vi "Depth Parser.vi"(8 "error in (no error)":errorcluster, 10 "RDS Serial Frame":refnum<class "RDS Serial Frame.lvclass">, 11 "Depth Instrument in":refnum<class "Depth Instrument.lvclass">) -> (0 "error out":errorcluster, 3 "Depth Instrument out":refnum<class "Depth Instrument.lvclass">)   [LabVIEW 2015, in "Depth Instrument.lvlib" / "Depth Instrument.lvclass"]
uses:
  Depth Instrument.lvclass
  Libraries/RDS Serial Handler/RDS Serial Frame.lvclass
  Libraries/RDS Child Messages/AIP Status Message/AIP Status Response.lvclass
  Libraries/RDS Instruments/AIP/AIP Status.ctl
  Libraries/RDS Instruments/AIP/AIP States.ctl
  Libraries/RDS Serial Handler/RDS Serial Frame.lvclass/RDS Serial Frame.ctl
  Libraries/RDS Framework/RDS Message ID.ctl
  Libraries/RDS Child Messages/Depth Data Message/Depth Data Message.lvclass
  Libraries/RDS Child Messages/Depth Data Message/Depth Data.ctl
  Depth Instrument.lvclass/Depth Instrument.ctl
  Libraries/RDS Framework/RDS Message Class/RDS Message.lvclass/RDS Message.ctl
  Libraries/RDS Child Messages/Depth Data Message/Depth Data Message.lvclass/Depth Data Message.ctl
  Libraries/RDS Serial Handler/RDS Serial Handler.lvlib
  Libraries/RDS Instruments/RDS Instrument Library.lvlib
  Libraries/RDS Child Messages/RDS Child Messages.lvlib
  AIP Instrument/AIP Instrument/AIP Instrument.lvclass
  Libraries/RDS Framework/RDS Message Class/RDS Message.lvclass
  Actors/RDS Parent Actor/RDS Parent Actor/RDS Parent Actor.lvclass
panel:
  out "AIP State":T1
  out "AIP Status Response":refnum<class "AIP Status Response.lvclass">
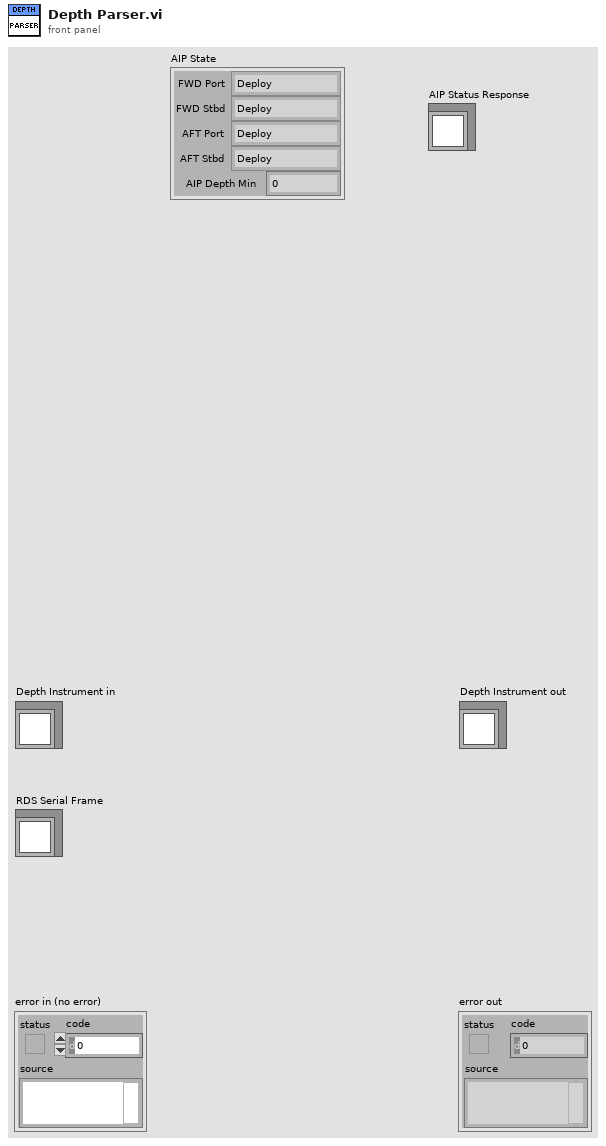
[diagram p1: front panel]
types:
  T1 = typedef "RDS Instrument Library.lvlib/AIP Status.ctl" = cluster{"FWD Port":T2, "FWD Stbd":T2, "AFT Port":T2, "AFT Stbd":T2, "AIP Depth Min":u8}
  T2 = typedef "RDS Instrument Library.lvlib/AIP States.ctl" = enum16{"Deploy", "Deploying", "Deployed", "Stow", "Stowing", "Stowed", "Fault", "brakeOnStow", "breakOnDeploy", "Stopped", "Stopping"}
  T3 = typedef "RDS Child Messages.lvlib/Depth Data.ctl" = cluster{"Depth":sgl, "Water Temp":i8}
  T4 = typedef "RDS Child Messages.lvlib/RDS Message ID.ctl" = enum16{"RDS Hello World", "String Message", "AIP_Status", "AIP_Command", "GPS_Data", "MCB_Command", "MCB_Status", "Compass_Data", "Depth_Data", "Battery_Data", "Contoller_State", "Set_Mag_Dev", "BTB_Shutdown", "State_Sample_Request", "State_Sample", "PID_Gains_Set", "Helm_Limiter_Set", "Helm_Heading_Command", "Helm_Steering_Command", "Helm_Status", "Controller_Message", "AIP_Set_Min_Depth", "Mission_Controller_State", "Mission_Upload", "Mission_Set_Op_and_Run", "Mission_Settings_Set"}
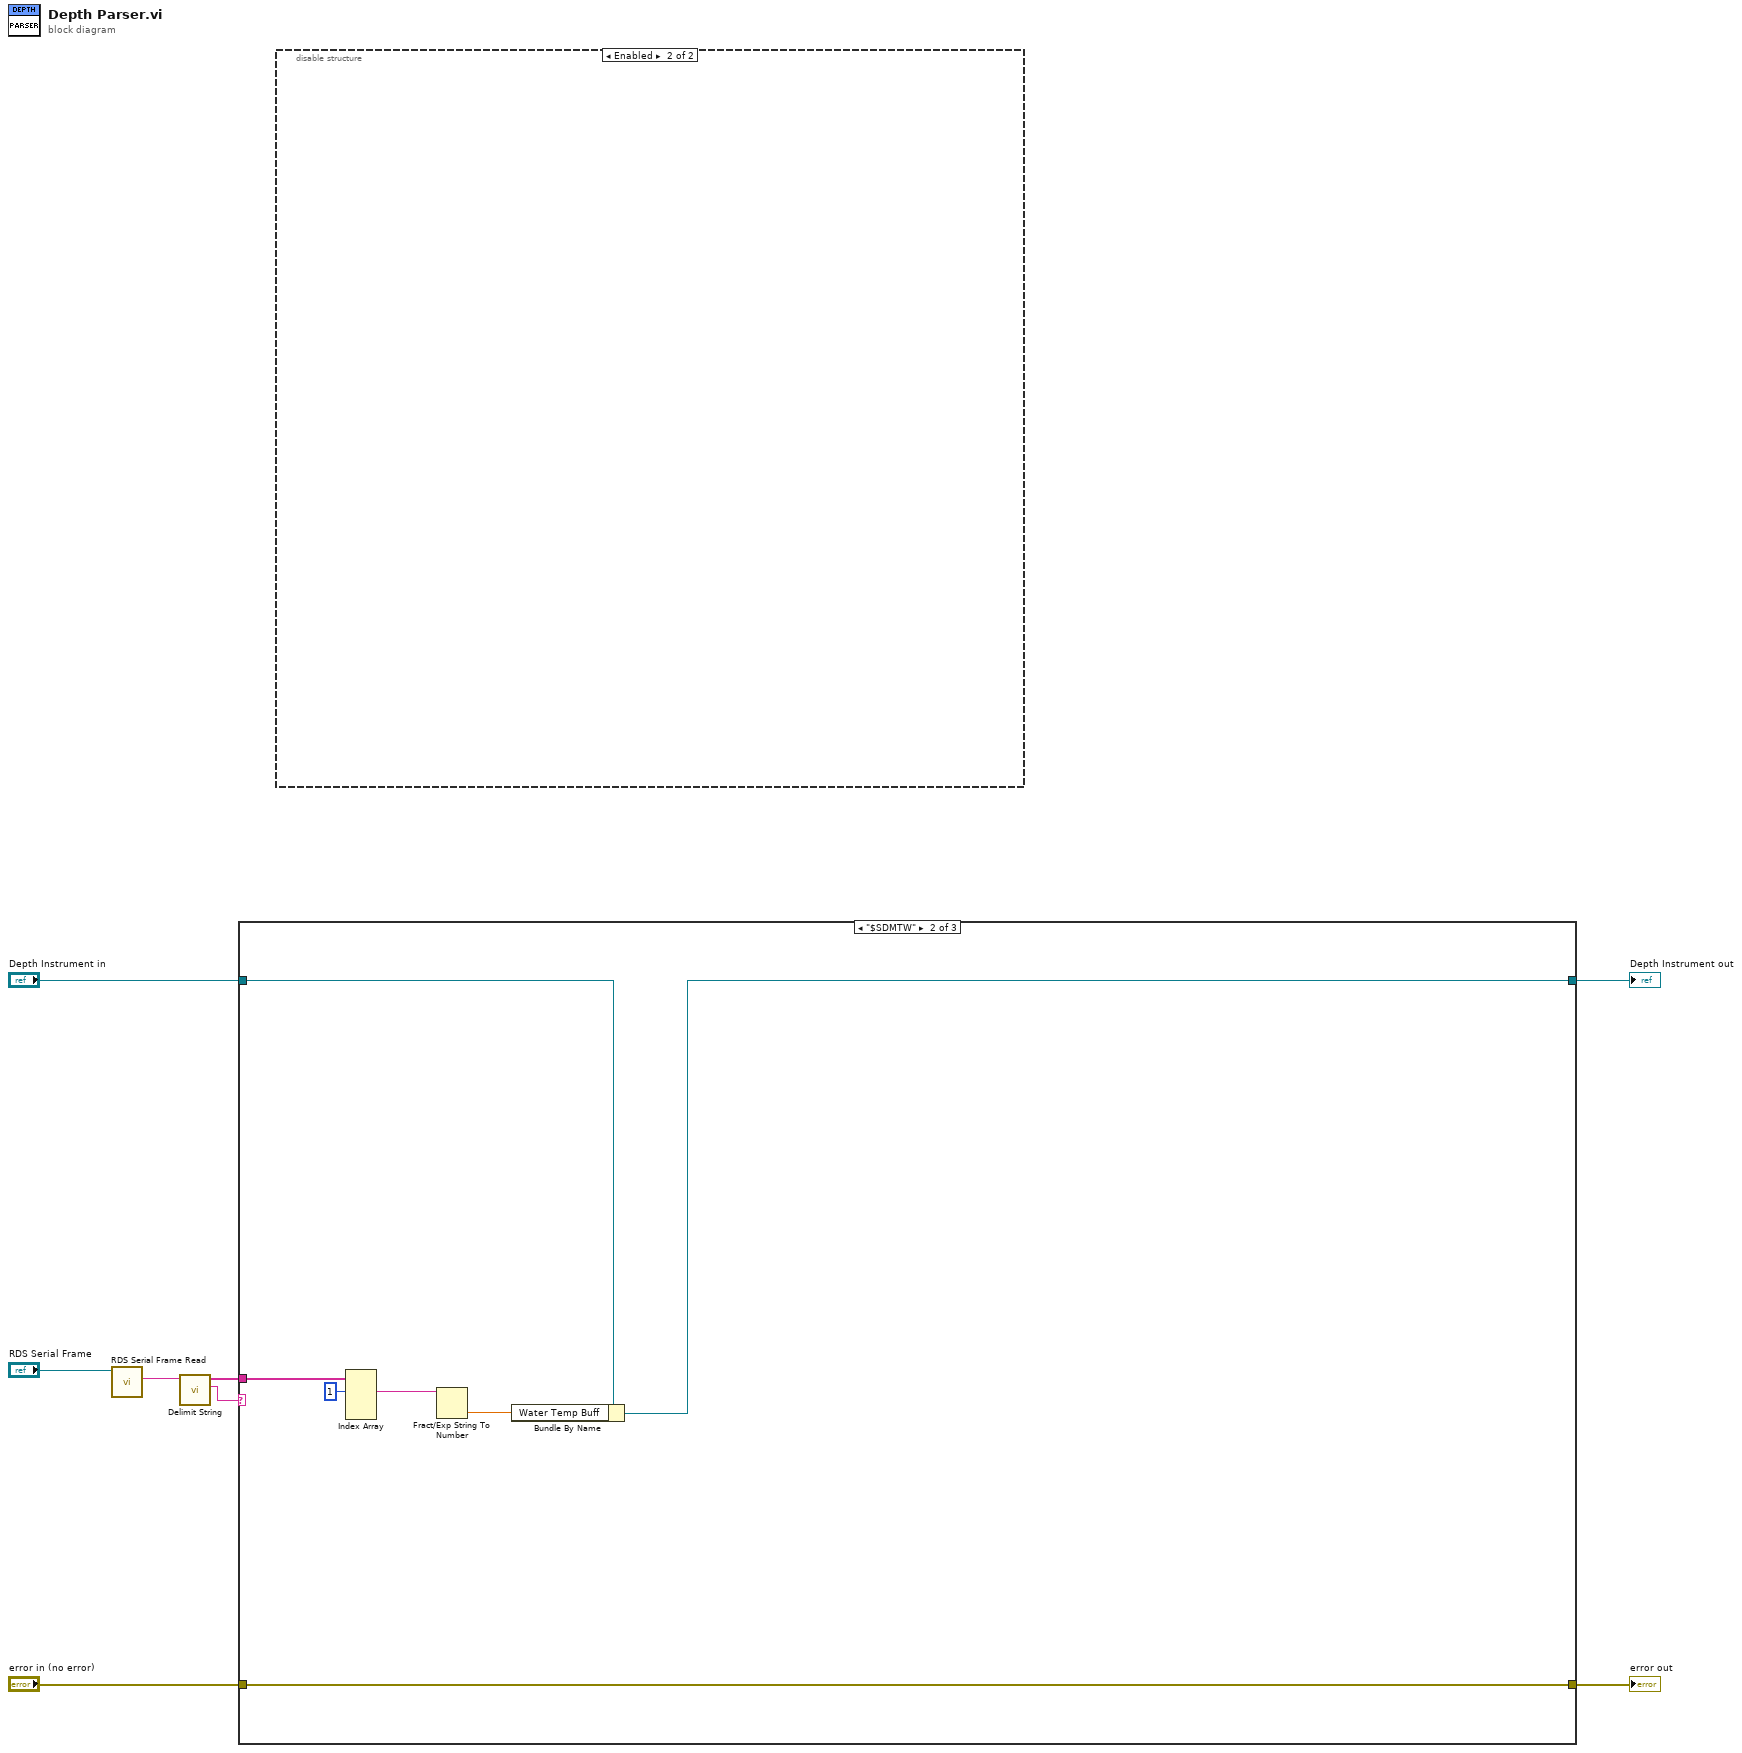
[diagram p0: block diagram]
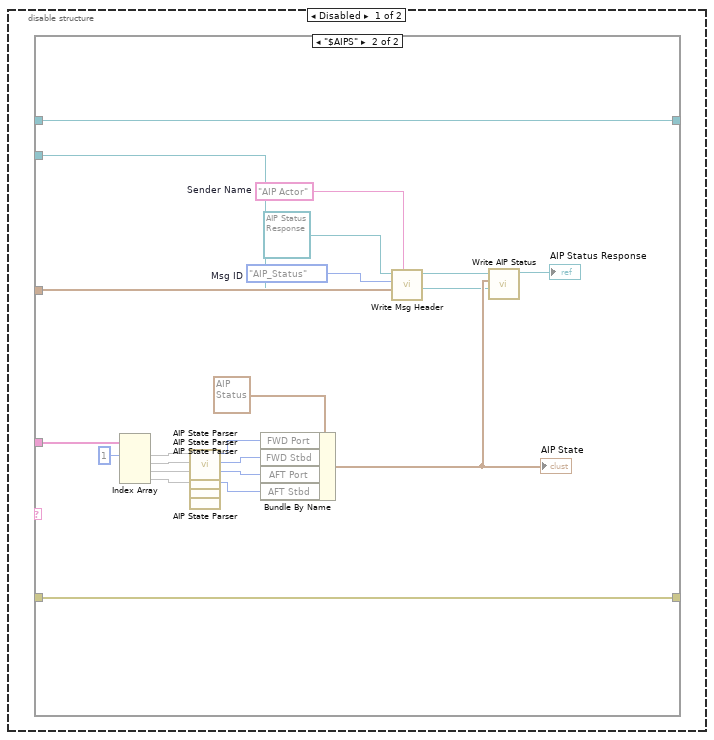
[diagram p2: hidden frame]
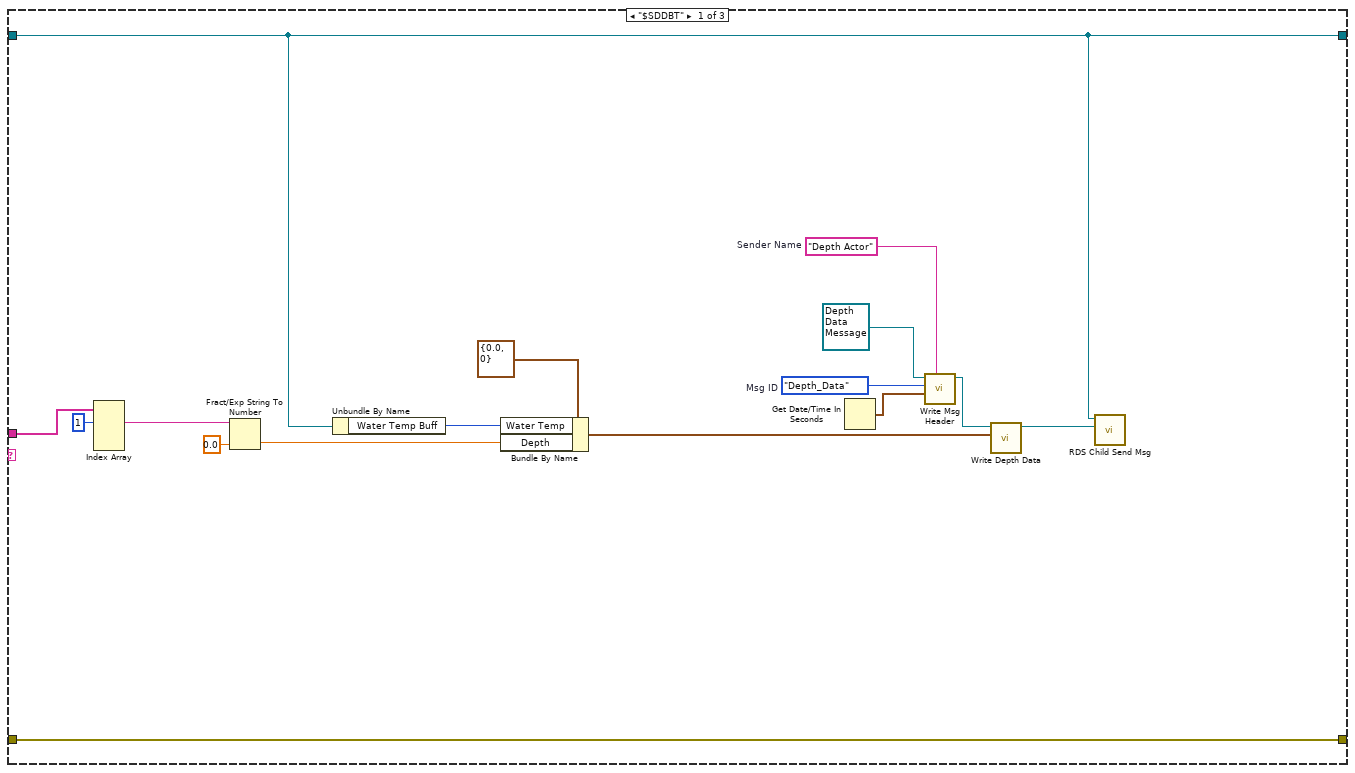
[diagram p4: hidden frame]
diagram:
  n1 = call "RDS Serial Frame Read.vi"("RDS Serial Frame in"="RDS Serial Frame") -> ("Serial String"=w1:string)  [unwired: 7 in, 3 out]
  n2 = call "Delimit String.vi"("Serial String"=w1) -> ("First Element"=w4:string, "All Elements"=w5:string[])  [unwired: 9 in]
  n3 = case shown="\"$SDMTW\"" w4 {
    tunnel: [w22 w25 w32] -> w8
    tunnel: [w15 w26 w33] -> w6
    tunnel: "Depth Instrument in" -> [w15 w27 w33]
    tunnel: w5 -> [w23 w29 _]
    tunnel: "error in (no error)" -> [w22 w25 w32]
    frame "$SDDBT" {
      w20 = "Depth Actor"  # Sender Name
      w21 = RDS_Message_ID."Depth_Data"  # Msg ID
      n4 = Index Array(array=w23, index #1=1 ("index")) -> (element #1=w17:string)  [unwired: 3 in, 3 out]
      n5 = Fract/Exp String To Number(string=w17, default (0 dbl)=sgl 0.0 ("default (0 DBL)")) -> (number=w12:sgl)  [unwired: 2 in, 1 out]
      n6 = Unbundle By Name(w15) -> ("Water Temp Buff"=w13:i8)
      n7 = Bundle By Name(cluster=T3 {"Depth"=0.0, "Water Temp"=0} ("Depth Data"), "Water Temp"=w13, "Depth"=w12) -> (w11:T3)
      n8 = Get Date/Time In Seconds() -> (seconds since 1Jan1904=w10:timestamp)
      n9 = call "Write Msg Header.vi"("Sender Name"=w20, "Time Stamp"=w10, "Msg ID"=w21, "RDS Message in"=refnum<class "Depth Data Message.lvclass"> refnum ("RDS Child Messages.lvlib:Depth Data Message.lvclass")) -> ("RDS Message out"=w18:refnum<class "Depth Data Message.lvclass">)  [unwired: 6 in, 1 out]
      n10 = call "Write Depth Data.vi"("Depth Data"=w11, "Depth Data Message in"=w18) -> ("Depth Data Message out"=w16:refnum<class "Depth Data Message.lvclass">)  [unwired: 8 in, 1 out]
      n11 = call "RDS Child Send Msg.vi"("RDS Message"=w16, "RDS Parent Actor in"=w15) -> ()  [unwired: 8 in, 2 out]
    }
    frame "$SDMTW" {
      n12 = Index Array(array=w29, index #1=1 ("index")) -> (element #1=w30:string)  [unwired: 3 in, 3 out]
      n13 = Fract/Exp String To Number(string=w30) -> (number=w28:dbl)  [unwired: 3 in, 1 out]
      n14 = Bundle By Name(cluster=w27, "Water Temp Buff"=w28) -> (w26:refnum<class "Depth Instrument.lvclass">)
    }
    frame "Error", Default {
    }
  }
  "error out" <- w8
  "Depth Instrument out" <- w6
  n15 = disable-structure shown="Enabled" {
    frame Disabled {
      n16 = case shown="\"$AIPS\"" {
        selector: _ -> [_ _]
        tunnel: _ -> [_ w56]
        tunnel: _ -> [_ w44]
        tunnel: _ -> [_ w39]
        tunnel: [w35 w37] -> _
        tunnel: _ -> [w35 w37]
        tunnel: [w34 w36] -> _
        tunnel: _ -> [w34 w36]
        frame "False", Default {
        }
        frame "$AIPS" {
          w42 = "AIP Actor"  # Sender Name
          w43 = RDS_Message_ID."AIP_Status"  # Msg ID
          n17 = Index Array(array=w56, index #1=1 ("index")) -> (element #1=w55, element #2=w54, element #3=w53, element #4=w52)  [unwired: 3 in]
          n18 = call "AIP State Parser.vi"("String"=w55) -> ("AIP States"=w50:T2)  [unwired: 8 in]
          n19 = call "AIP State Parser.vi"("String"=w54) -> ("AIP States"=w49:T2)  [unwired: 8 in]
          n20 = call "AIP State Parser.vi"("String"=w53) -> ("AIP States"=w48:T2)  [unwired: 8 in]
          n21 = call "AIP State Parser.vi"("String"=w52) -> ("AIP States"=w47:T2)  [unwired: 8 in]
          n22 = Bundle By Name(cluster=T1 {"FWD Port"=enum."Deploy", "FWD Stbd"=enum."Deploy", "AFT Port"=enum."Deploy", "AFT Stbd"=enum."Deploy", "AIP Depth Min"=0} ("AIP Status"), "FWD Port"=w50, "FWD Stbd"=w49, "AFT Port"=w48, "AFT Stbd"=w47) -> (w40:T1)
          "AIP State" <- w40
          n23 = call "Write Msg Header.vi"("Sender Name"=w42, "Time Stamp"=w44, "Msg ID"=w43, "RDS Message in"=refnum<class "AIP Status Response.lvclass"> refnum ("RDS Child Messages.lvlib:AIP Status Response.lvclass")) -> ("RDS Message out"=w41:refnum<class "AIP Status Response.lvclass">)  [unwired: 6 in, 1 out]
          n24 = call "Write AIP Status.vi"("Raw Frame"=w39, "AIP Status"=w40, "AIP Status Response in"=w41) -> ("AIP Status Response out"=→"AIP Status Response":refnum<class "AIP Status Response.lvclass">)  [unwired: 7 in, 1 out]
        }
      }
    }
    frame Enabled {
    }
  }
